vi "VecBuilder_7x1Fill.vi"(5 "R0":dbl, 6 "R6":dbl, 7 "R1":dbl, 8 "R5":dbl, 9 "R4":dbl, 10 "R3":dbl, 11 "R2":dbl) -> (3 "output matrix":T1)   [LabVIEW 2019, in "Trajectory_Library.lvlib"]
doc: "Build a 7 x 1 Matrix (vector) from an array of input values.\n\nInputs:\n -- R0 -- Input value 1\n -- R1 -- Input value 2\n -- R2 -- Input value 3\n -- R3 -- Input value 4\n -- R4 -- Input value 5\n -- R5 -- Input value 6\n -- R6 -- Input value 7\n\nOutputs:\n -- Output Matrix -- Resulting 7 x 1 matrix (vector)"
uses:
  Trajectory_Library.lvlib
  <vilib>/Analysis/Matrix/Datatypes/RealMatrix.ctl
  <vilib>/Analysis/Matrix/NI_Matrix.lvlib
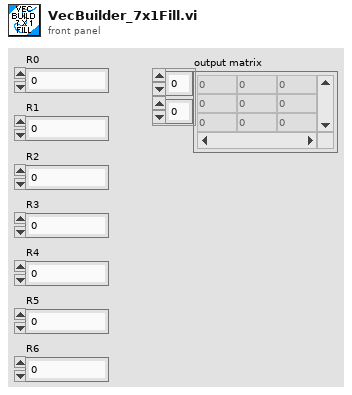
[diagram p1: front panel]
types:
  T1 = typedef "NI_Matrix.lvlib/RealMatrix.ctl" = dbl[][]
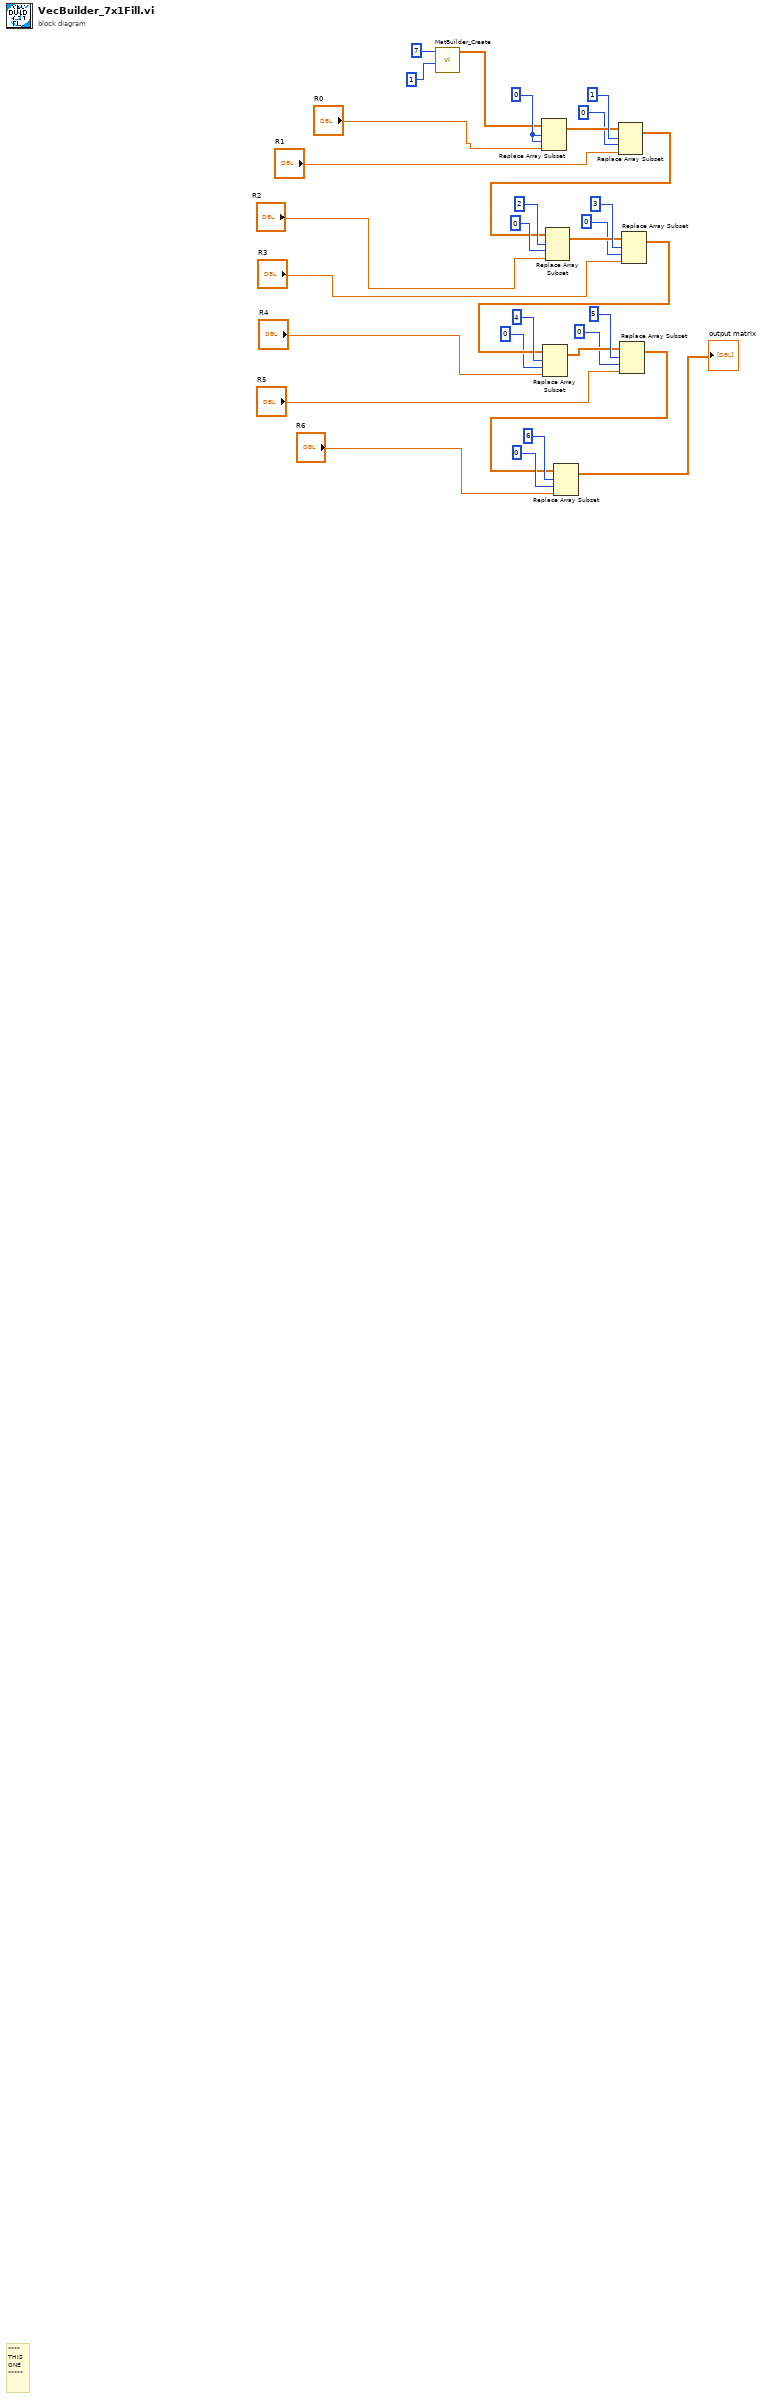
[diagram p0: block diagram]
diagram:
  w14 = 0 ("index (col)")
  # "****\nTHIS\nONE\n*****"
  n1 = call "MatBuilder_Create.vi"("Columns"=1, "Rows"=7) -> ("output matrix"=w6:T1)  [unwired: 9 in]
  n2 = Replace Array Subset(array=w6, new element="R0", index (row)=w14, index (col)=w14) -> (w12:T1)
  n3 = Replace Array Subset(array=w12, new element="R1", index (row)=1 ("index (col)"), index (col)=0 ("disabled index (col)")) -> (w7:T1)
  n4 = Replace Array Subset(array=w7, new element="R2", index (row)=2 ("index (col)"), index (col)=0 ("disabled index (col)")) -> (w28:T1)
  n5 = Replace Array Subset(array=w28, new element="R3", index (row)=3 ("index (col)"), index (col)=0 ("disabled index (col)")) -> (w20:T1)
  n6 = Replace Array Subset(array=w20, new element="R4", index (row)=4 ("index (col)"), index (col)=0 ("disabled index (col)")) -> (w19:T1)
  n7 = Replace Array Subset(array=w19, new element="R5", index (row)=5 ("index (col)"), index (col)=0 ("disabled index (col)")) -> (w3:T1)
  n8 = Replace Array Subset(array=w3, new element="R6", index (row)=6 ("index (col)"), index (col)=0 ("disabled index (col)")) -> (→"output matrix":T1)
